vi "encode_url_parameters.vi"(8 "error in (no error)":errorcluster, 10 "value []":string[](array[string]), 11 "key []":string[](array[string])) -> (0 "error out":errorcluster, 3 "url_encoded_string":string)   [LabVIEW 2015, in "lv-dropbox.lvlib"]
uses:
  lv-dropbox.lvlib
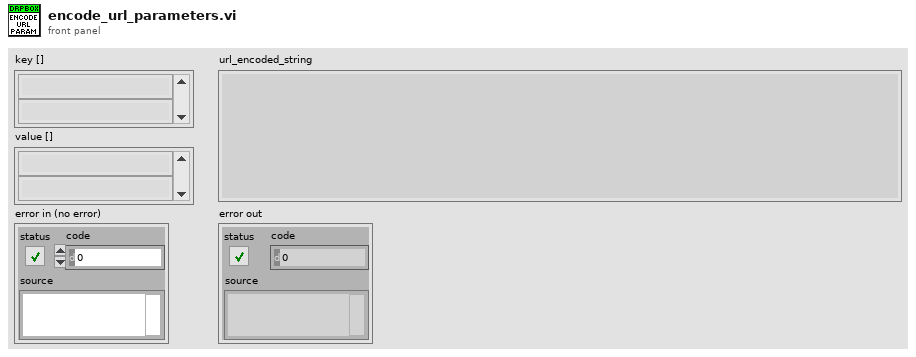
[diagram p1: front panel]
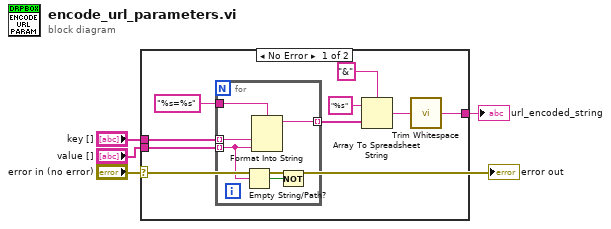
[diagram p0: block diagram]
diagram:
  n1 = case shown="No Error" "error in (no error)" {
    tunnel: "key []" -> [w12 _]
    tunnel: "value []" -> [w11 _]
    tunnel: [w5 _] -> w2
    frame No Error {
      n2 = for {
        tunnel: w12 -> [w17] mode=indexing
        tunnel: w11 -> [w14] mode=indexing
        tunnel: "%s=%s" ("format string") -> [w16]
        tunnel: [w15] -> w9 mode=indexing
        n3 = Empty String/Path?(string/path=w14) -> (empty?=w13:bool)
        n4 = Format Into String(format string=w16, w17, w14) -> (resulting string=w15:string)  [unwired: 2 in, 1 out]
        n5 = Not(x=w13) -> ()  [unwired: 1 out]
      }
      n6 = Array To Spreadsheet String(delimiter (Tab)="&", array=w9, 3:"%s" ("format string")) -> (spreadsheet string=w6:string)
      n7 = call <vilib>:"Trim Whitespace.vi"("string"=w6) -> ("trimmed string"=w5:string)  [unwired: 1 in]
    }
    frame Error {
    }
  }
  "url_encoded_string" <- w2
  "error out" <- "error in (no error)"
